vi "6500电流加载及换向回读.vi"(0 "2700 in":refnum<visa-resource-name>, 1 "IT6512C in":refnum<visa-resource-name>, 2 "输入电流":dbl, 3 "Delay Time (s)":dbl=0.3 caption="延迟时间(s)", 5 "error in":errorcluster) -> (14 "2700 out":refnum<visa-resource-name>, 15 "IT6512C out":refnum<visa-resource-name>, 16 "实际电流":dbl, 19 "error out":errorcluster)   [LabVIEW 2020]
uses:
  <vilib>/Modbus/master/Modbus Master.lvclass
  D/Program Files (x86)/National Instruments/LabVIEW 2020/instr.lib/Keithley 27XX/Public/Data/Read Multiple Direct.vi
  D/Program Files (x86)/National Instruments/LabVIEW 2020/instr.lib/IT6500/IT6500.lvlib
  D/Program Files (x86)/National Instruments/LabVIEW 2020/instr.lib/Keithley 27XX/Keithley 27XX.lvlib
panel:
  in  "Modbus master in":refnum<class "Modbus Master.lvclass"> caption="Modbus主设备输入"
  # "IT6512C 电流加载及换向"
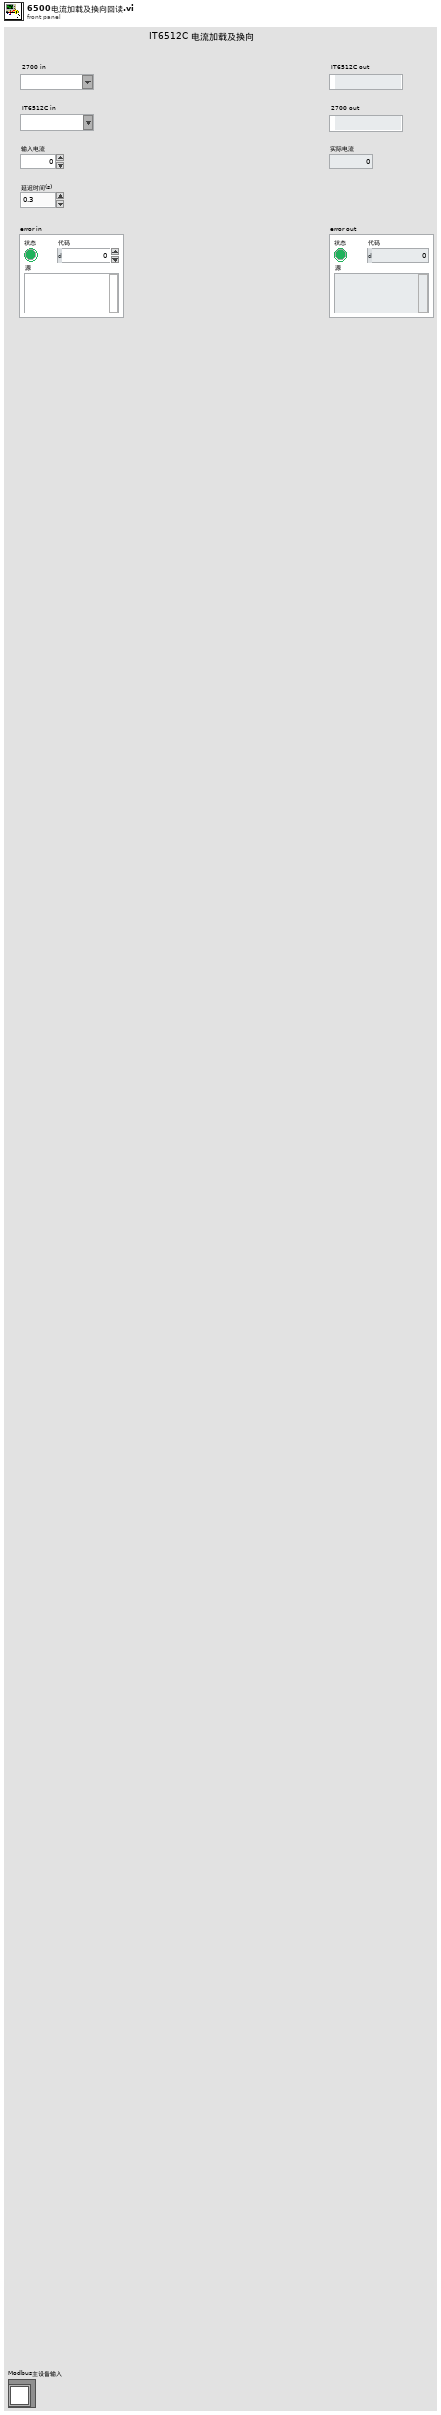
[diagram p1: front panel]
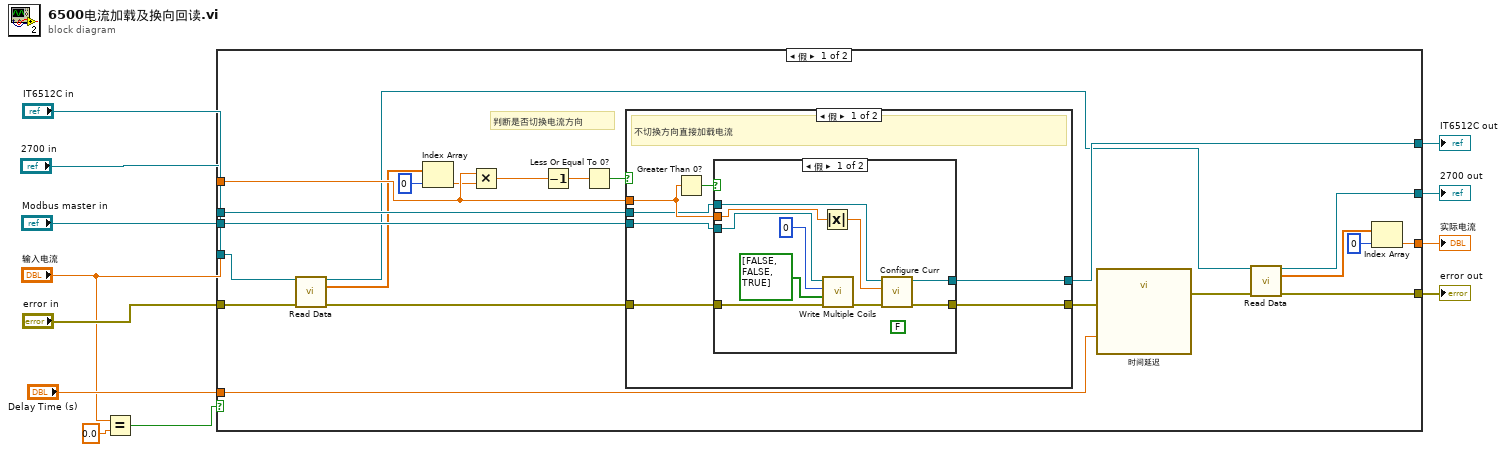
[diagram p0: block diagram]
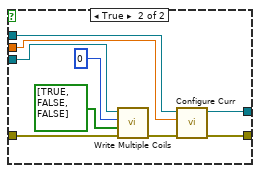
[diagram p2: hidden frame]
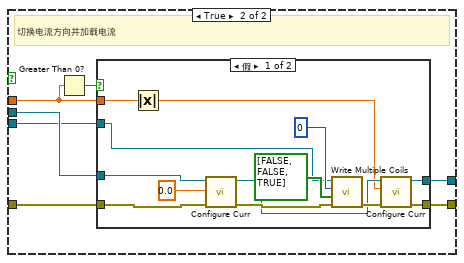
[diagram p3: hidden frame]
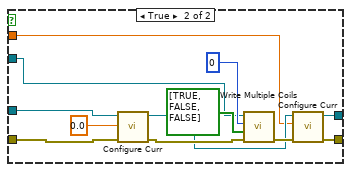
[diagram p4: hidden frame]
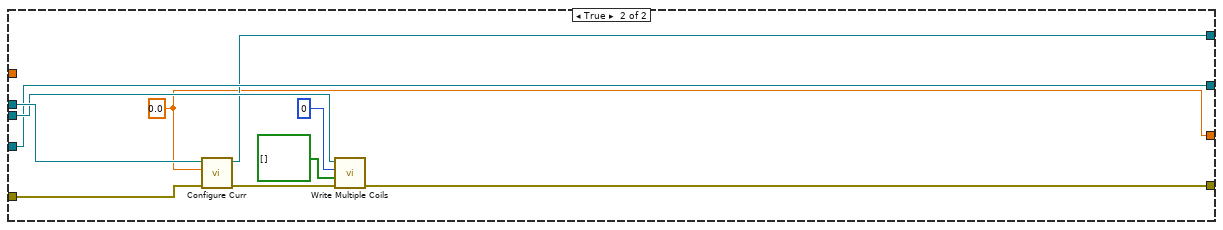
[diagram p5: hidden frame]
diagram:
  n1 = Equal?(x="输入电流", y=0.0) -> (x = y?=w2:bool)
  n2 = case shown="假" w2 {
    tunnel: "IT6512C in" -> [w31 w102]
    tunnel: "Modbus master in" -> [w30 w100]
    tunnel: [w14 w94] -> w10
    tunnel: "Delay Time (s)" -> [w28 _]
    tunnel: "error in" -> [w24 w95]
    tunnel: [w27 w96] -> w7
    tunnel: "2700 in" -> [w25 w97]
    tunnel: [w15 w97] -> w5
    tunnel: "输入电流" -> [w26 _]
    tunnel: [w17 w93] -> w1
    frame False {
      # "判断是否切换电流方向"
      n3 = call-poly "Read Data.vi"("VISA resource name"=w25, "error in (no error)"=w24) -> ("VISA resource name out"=w18:refnum<visa-resource-name>, "Measurement Data"=w22:dbl[], "error out"=w23:errorcluster)  [unwired: 8 in, 3 out]
      n4 = Index Array(array=w22, index=0 ("索引")) -> (element=w13:dbl)
      n5 = Multiply(x=w26, y=w13) -> (x*y=w33:dbl)
      n6 = Decrement(x=w33) -> (x-1=w32:dbl)
      n7 = Less Or Equal To 0?(x=w32) -> (x <= 0?=w34:bool)
      n8 = case shown="假" w34 {
        tunnel: w26 -> [w40 w67]
        tunnel: w23 -> [w37 w62]
        tunnel: w31 -> [w39 w65]
        tunnel: w30 -> [w35 w64]
        tunnel: [w38 w63] -> w29
        tunnel: [w36 w61] -> w27
        frame False {
          # "不切换方向直接加载电流"
          n9 = Greater Than 0?(x=w40) -> (x > 0?=w41:bool)
          n10 = case shown="假" w41 {
            tunnel: w40 -> [w51 w60]
            tunnel: w39 -> [w49 w59]
            tunnel: [w48 w58] -> w38
            tunnel: w37 -> [w45 w52]
            tunnel: [w47 w57] -> w36
            tunnel: w35 -> [w44 w55]
            frame False {
              (unwired) FALSE ("Boolean")
              n11 = Absolute Value(x=w51) -> (abs(x)=w50:dbl)
              n12 = call-dynamic "Write Multiple Coils.vi"("error in (no error)"=w45, "coil values"=bool[] [FALSE, FALSE, TRUE], "starting address"=u16 0, "Modbus master in"=w44) -> ("error out"=w43:errorcluster)  [unwired: 6 in, 1 out]
              n13 = call "Configure Curr.vi"("error in (no error)"=w43, "Curr(0)"=w50, "VISA resource name"=w49) -> ("error out"=w48:errorcluster, "VISA resource name out"=w47:refnum<visa-resource-name>)  [unwired: 7 in]
            }
            frame True {
              n14 = call-dynamic "Write Multiple Coils.vi"("error in (no error)"=w52, "coil values"=bool[] [TRUE, FALSE, FALSE], "starting address"=u16 0, "Modbus master in"=w55) -> ("error out"=w56:errorcluster)  [unwired: 6 in, 1 out]
              n15 = call "Configure Curr.vi"("error in (no error)"=w56, "Curr(0)"=w60, "VISA resource name"=w59) -> ("error out"=w58:errorcluster, "VISA resource name out"=w57:refnum<visa-resource-name>)  [unwired: 7 in]
            }
          }
        }
        frame True {
          # "切换电流方向并加载电流"
          n16 = Greater Than 0?(x=w67) -> (x > 0?=w66:bool)
          n17 = case shown="假" w66 {
            tunnel: w67 -> [w74 w86]
            tunnel: w65 -> [w72 w83]
            tunnel: w64 -> [w71 w85]
            tunnel: [w70 w84] -> w63
            tunnel: w62 -> [w69 w82]
            tunnel: [w68 w81] -> w61
            frame False {
              n18 = Absolute Value(x=w74) -> (abs(x)=w73:dbl)
              n19 = call "Configure Curr.vi"("error in (no error)"=w69, "Curr(0)"=0.0, "VISA resource name"=w72) -> ("error out"=w77:errorcluster, "VISA resource name out"=w75:refnum<visa-resource-name>)  [unwired: 7 in]
              n20 = call-dynamic "Write Multiple Coils.vi"("error in (no error)"=w77, "coil values"=bool[] [FALSE, FALSE, TRUE], "starting address"=u16 0, "Modbus master in"=w71) -> ("error out"=w76:errorcluster)  [unwired: 6 in, 1 out]
              n21 = call "Configure Curr.vi"("error in (no error)"=w76, "Curr(0)"=w73, "VISA resource name"=w75) -> ("error out"=w70:errorcluster, "VISA resource name out"=w68:refnum<visa-resource-name>)  [unwired: 7 in]
            }
            frame True {
              n22 = call "Configure Curr.vi"("error in (no error)"=w82, "Curr(0)"=0.0, "VISA resource name"=w83) -> ("error out"=w89:errorcluster, "VISA resource name out"=w87:refnum<visa-resource-name>)  [unwired: 7 in]
              n23 = call-dynamic "Write Multiple Coils.vi"("error in (no error)"=w89, "coil values"=bool[] [TRUE, FALSE, FALSE], "starting address"=u16 0, "Modbus master in"=w85) -> ("error out"=w88:errorcluster)  [unwired: 6 in, 1 out]
              n24 = call "Configure Curr.vi"("error in (no error)"=w88, "Curr(0)"=w86, "VISA resource name"=w87) -> ("error out"=w84:errorcluster, "VISA resource name out"=w81:refnum<visa-resource-name>)  [unwired: 7 in]
            }
          }
        }
      }
      n25 = call "时间延迟"("error in (no error)"=w29, "Delay Time (s)"=w28) -> ("error out"=w16:errorcluster)  [unwired: 9 in]
      n26 = call-poly "Read Data.vi"("VISA resource name"=w18, "error in (no error)"=w16) -> ("VISA resource name out"=w15:refnum<visa-resource-name>, "Measurement Data"=w19:dbl[], "error out"=w14:errorcluster)  [unwired: 8 in, 3 out]
      n27 = Index Array(array=w19, index=0 ("索引")) -> (element=w17:dbl)
    }
    frame True {
      w93 = 0.0 ("Curr(0)")
      n28 = call "Configure Curr.vi"("error in (no error)"=w95, "Curr(0)"=w93, "VISA resource name"=w102) -> ("error out"=w101:errorcluster, "VISA resource name out"=w96:refnum<visa-resource-name>)  [unwired: 7 in]
      n29 = call-dynamic "Write Multiple Coils.vi"("error in (no error)"=w101, "coil values"=bool[] [], "starting address"=u16 0, "Modbus master in"=w100) -> ("error out"=w94:errorcluster)  [unwired: 6 in, 1 out]
    }
  }
  "error out" <- w10
  "实际电流" <- w1
  "IT6512C out" <- w7
  "2700 out" <- w5
